vi "Compiler.vi"(7 "Sequence folder path":path, 8 "error in (no error)":errorcluster, 9 "Message Priority(Normal)":T1=enum."Normal", 10 "Override Look up table":variant, 11 "Uncompiled sequence in":T2[](array[typedef])) -> (0 "error out":errorcluster, 1 "Success?":bool, 3 "Batch Msg out":refnum<class "Batch Msg.lvclass">)   [LabVIEW 2020, in "Sequencer.lvlib"]
doc: "Compile an uncompiled sequence into a Batch Msg."
uses:
  Sequencer.lvlib
  Controls/Ctl_SequenceElement.ctl
  Controls/Ctl_SequenceControlElement.ctl
  PPL/HDH.Actor Framework.Core.Msg.lvlibp/Flex Msg/Controls/Ctl_Control Element.ctl
  Sequencer Messages/Batch Msg/Batch Msg.lvclass
  C:/Current projects/WS/LV32.2020..HDH.ActorFramework.Core/Actor/Sequencer/Sequencer Messages/Sequencer Msg/Sequencer Msg.lvclass
  PPL/HDH.Actor Framework.Core.Actor.lvlibp/1abvi3w/vi.lib/ActorFramework/Message Enqueuer/Message Priority.ctl
  Sequencer Messages/Batch Msg/Batch Msg.lvclass/Batch Msg.ctl
  Sequencer Messages/Sequencer Msg/Sequencer Msg.lvclass/Sequencer Msg.ctl
  Sequencer Messages/Sequencer Msg/Sequencer Msg.lvclass
  PPL/HDH.Actor Framework.Core.Msg.lvlibp
  PPL/HDH.Actor Framework.Core.Actor.lvlibp/1abvi3w/vi.lib/ActorFramework/Message Enqueuer/Message Enqueuer.lvclass
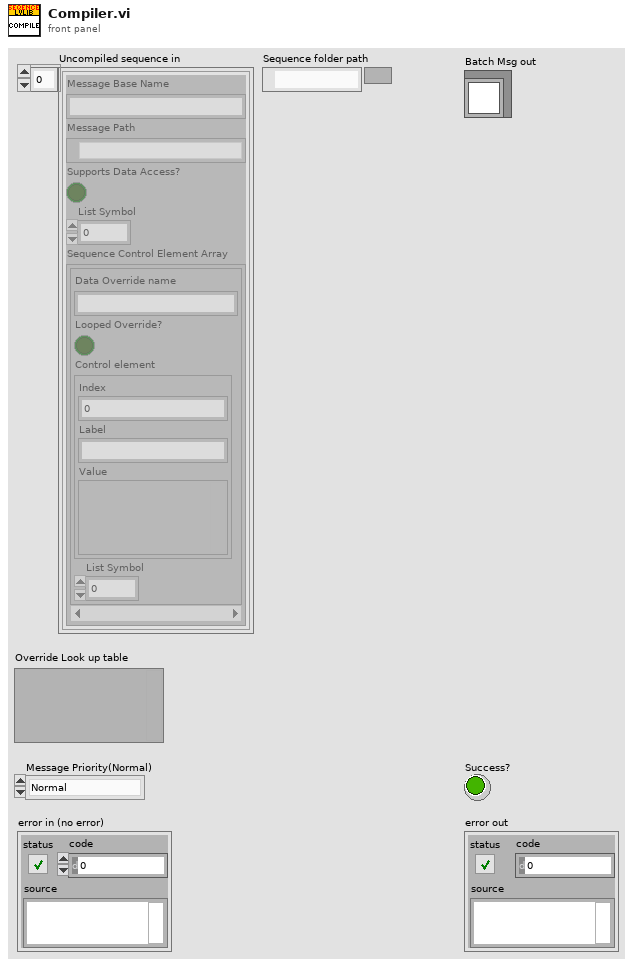
[diagram p1: front panel]
types:
  T1 = typedef "HDH.Actor Framework.Core.Actor.lvlibp/Message Enqueuer.lvclass/Message Priority.ctl" = enum16{"Low", "Normal", "High"}
  T2 = typedef "Sequencer.lvlib/Ctl_SequenceElement.ctl" = cluster{"Message Base Name":string, "Message Path":path, "Supports Data Access?":bool, "List Symbol":i32, "Sequence Control Element Array":T3[]}
  T3 = typedef "Sequencer.lvlib/Ctl_SequenceControlElement.ctl" = cluster{"Data Override name":string, "Looped Override?":bool, "Control element":T4, "List Symbol":i32}
  T4 = typedef "HDH.Actor Framework.Core.Msg.lvlibp/Ctl_Control Element.ctl" = cluster{"Index":i32, "Label":string, "Value":variant}
  T5 = typedef "Sequencer.lvlib/Ctl_MessageListElement.ctl" = cluster{"Base Name":string, "List index":i32, "Msg path":path, "Supports DA?":bool, "Symbol":i32}
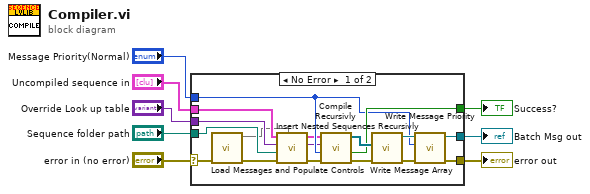
[diagram p0: block diagram]
diagram:
  n1 = case shown="No Error" "error in (no error)" {
    selector: "error in (no error)" -> [w11 w26]
    tunnel: "Override Look up table" -> [w14 _]
    tunnel: "Uncompiled sequence in" -> [w12 _]
    tunnel: "Message Priority(Normal)" -> [w18 _]
    tunnel: [w21 _] -> w4
    tunnel: [w20 w26] -> w3
    tunnel: [w19 _] -> w2
    tunnel: "Sequence folder path" -> [w13 _]
    frame No Error {
      n2 = call "Load Messages and Populate Controls.vi"("error in (no error)"=w11) -> ("error out"=w10:errorcluster, "Message map"=w9:map{string, T5})  [unwired: 9 in]
      n3 = call "Insert Nested Sequences Recursivly.vi"("Message map"=w9, "error in (no error)"=w10, "Sequence folder path"=w13, "Override Look up table in"=w14, "Uncompiled sequence in"=w12) -> ("error out"=w16:errorcluster, "Override Look up table out"=w15:variant, "Uncompiled Sequence out"=w17:T2[])  [unwired: 4 in]
      n4 = call "Compile Recursivly.vi"("error in (no error)"=w16, "Message Priority"=w18, "Override Look up table"=w15, "Uncompiled sequence in"=w17) -> ("error out"=w24:errorcluster, "Success?"=w19:bool, "Compiled Message Array"=w25:refnum<class "Message.lvclass">[])  [unwired: 4 in, 1 out]
      n5 = call "Write Message Array.vi"("error in (no error)"=w24, "Message Array"=w25) -> ("error out"=w22:errorcluster, "Batch Msg out"=w23:refnum<class "Batch Msg.lvclass">)  [unwired: 8 in]
      n6 = call "Write Message Priority.vi"("error in (no error)"=w22, "Priority"=w18, "Sequencer Msg in"=w23) -> ("error out"=w20:errorcluster, "Sequencer Msg out"=w21:refnum<class "Batch Msg.lvclass">)  [unwired: 7 in]
    }
    frame Error {
    }
  }
  "error out" <- w3
  "Success?" <- w2
  "Batch Msg out" <- w4
